vi "Execute.vi"(8 "error in (no error)":errorcluster, 9 "Consumer Queues in":T2, 10 "Trig Process Command in":refnum<class "Exit TRIG.lvclass">, 11 "Trig Process Data in":T1) -> (0 "error out":errorcluster, 1 "Consumer Queues out":T2, 2 "Stop?":bool, 3 "Trig Process Data out":T1)   [LabVIEW 2019, in "Trig Process.lvlib" / "Exit TRIG.lvclass"]
uses:
  Exit TRIG.lvclass
  TS Framework/Consumer Queues.ctl
  UI Process/Generic UI Command/Generic UI Process Command.lvclass
  DAC Process/Generic DAC Command/Generic DAC Process Command.lvclass
  Generic Trig Command/Generic Trig Process Command.lvclass
  Trig Process Data.ctl
  TS Framework/TS Framework.lvlib
  Trig Process.lvlib
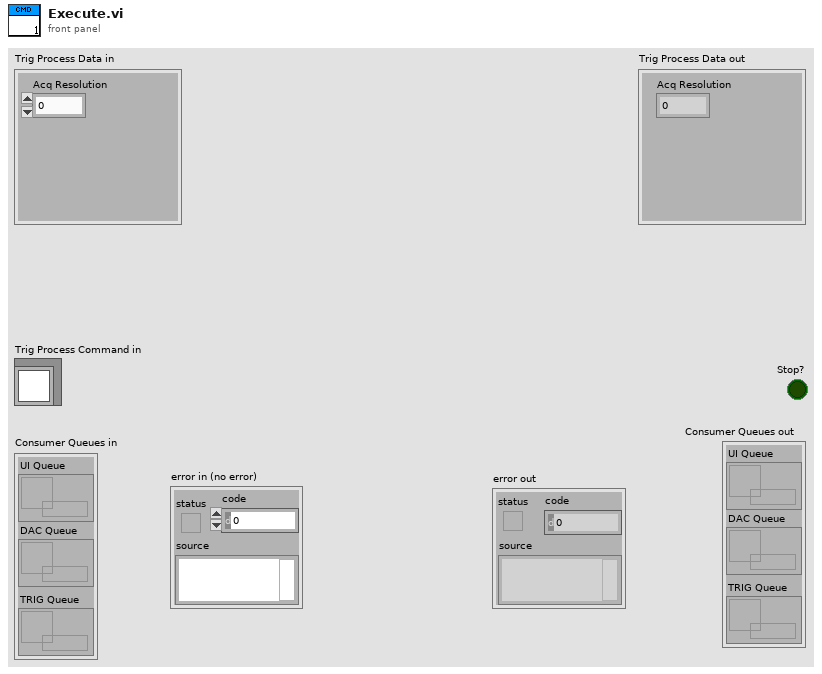
[diagram p1: front panel]
types:
  T1 = typedef "Trig Process.lvlib/Trig Process Data.ctl" = cluster{"Acq Resolution":u32}
  T2 = typedef "TS Framework.lvlib/Consumer Queues.ctl" = cluster{"UI Queue":refnum<queue>, "DAC Queue":refnum<queue>, "TRIG Queue":refnum<queue>}
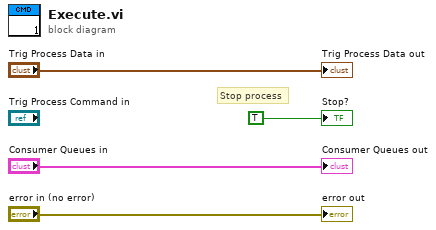
[diagram p0: block diagram]
diagram:
  # "Stop process"
  "error out" <- "error in (no error)"
  "Stop?" <- TRUE ("Stop?")
  "Consumer Queues out" <- "Consumer Queues in"
  "Trig Process Data out" <- "Trig Process Data in"
